vi "Write AppOutputData.vi"(8 "error in (no error)":errorcluster, 10 "AppOutputData":variant, 11 "RingdownPlugin in":refnum<class "RingdownPlugin.lvclass">) -> (0 "error out":errorcluster, 3 "RingdownPlugin out":refnum<class "RingdownPlugin.lvclass">)   [LabVIEW 2014, in "AppPlugins.lvlib" / "RingdownPlugin.lvclass"]
uses:
  RingdownPlugin.lvclass
  PublicAPI/TypeDef/RingdownOutput.ctl
  RingdownPlugin.lvclass/RingdownPlugin.ctl
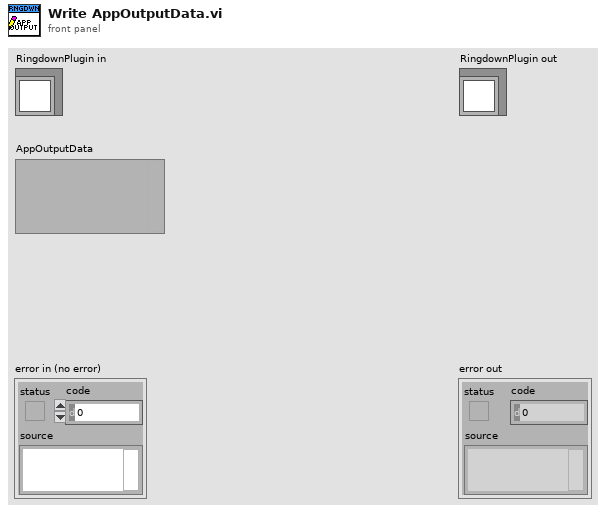
[diagram p1: front panel]
types:
  T1 = typedef "AppPlugins.lvlib/RingdownPlugin.lvclass/RingdownOutput.ctl" = cluster{"FramesPerSecond":dbl, "PronyEstimate":dbl[], "RingdownParameters":cluster{"Amplitude":dbl[], "Damping":dbl[], "Frequency":dbl[], "Phase":dbl[]}, "ReportingTime":dbl, "DataSize":u32, "InputSignal":dbl[]}
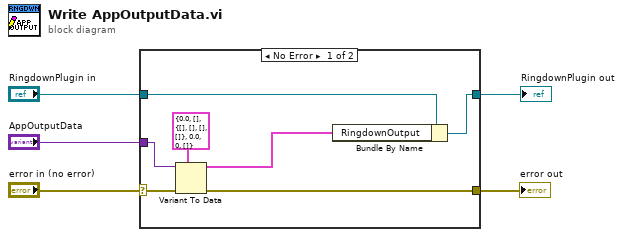
[diagram p0: block diagram]
diagram:
  n1 = case shown="No Error" "error in (no error)" {
    selector: "error in (no error)" -> [w11 w14]
    tunnel: [w6 w14] -> w4
    tunnel: "RingdownPlugin in" -> [w12 w13]
    tunnel: [w7 w13] -> w2
    tunnel: "AppOutputData" -> [w10 _]
    frame No Error {
      n2 = Variant To Data(error in=w11, type=T1 {"FramesPerSecond"=0.0, "PronyEstimate"=[], "RingdownParameters"={"Amplitude"=[], "Damping"=[], "Frequency"=[], "Phase"=[]}, "ReportingTime"=0.0, "DataSize"=0, "InputSignal"=[]} ("RingdownOutput"), Variant=w10) -> (data=w8:T1, error out=w6:errorcluster)
      n3 = Bundle By Name(cluster=w12, "RingdownOutput"=w8) -> (w7:refnum<class "RingdownPlugin.lvclass">)
    }
    frame Error {
    }
  }
  "error out" <- w4
  "RingdownPlugin out" <- w2
